vi "writeSummaryStateSV.vi"(8 "error in (no error)":errorcluster, 10 "componentStateValues":T1, 11 "ComponentData in":refnum<class "ComponentData.lvclass">) -> (0 "error out":errorcluster, 3 "ComponentData out":refnum<class "ComponentData.lvclass">)   [LabVIEW 2013, in "ComponentData.lvlib" / "ComponentData.lvclass"]
uses:
  <userlib>/Common/Component/Application/RT/ComponentData/ComponentData/ComponentData.lvclass
  <userlib>/Common/Component/Application/RT/ComponentData/componentStateValues.ctl
  <userlib>/Common/Component/Application/RT/ComponentData.lvlib
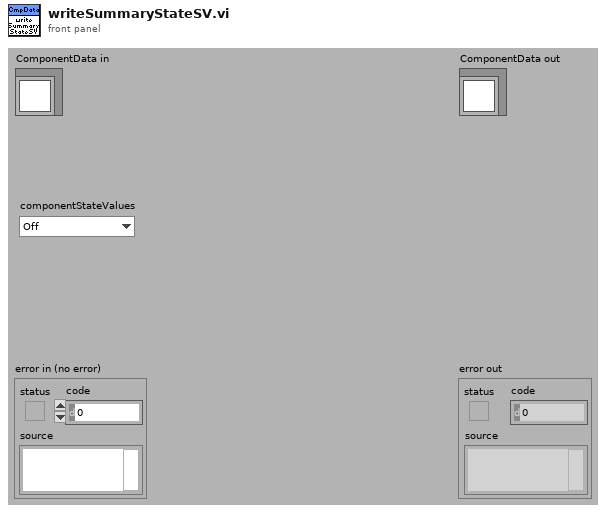
[diagram p1: front panel]
types:
  T1 = typedef "ComponentData.lvlib/componentStateValues.ctl" = enum16{"Off", "Standby", "Enabled", "Disabled", "Fault"}
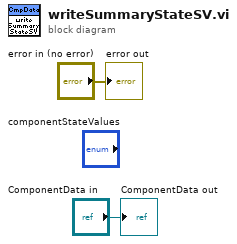
[diagram p0: block diagram]
diagram:
  "error out" <- "error in (no error)"
  "ComponentData out" <- "ComponentData in"
